vi "Initiate TS.vi"(8 "error in":errorcluster, 11 "HTS Test Stand in":refnum<class "HTS Test Stand.lvclass">) -> (0 "error out":errorcluster, 3 "HTS Test Stand out":refnum<class "HTS Test Stand.lvclass">)   [LabVIEW 2019, in "Test Stands.lvlib" / "HTS Test Stand.lvclass"]
uses:
  HTS Test Stand.lvclass
  DAC/HTS/Vacum Valve/DAC Vacum Valve.lvclass
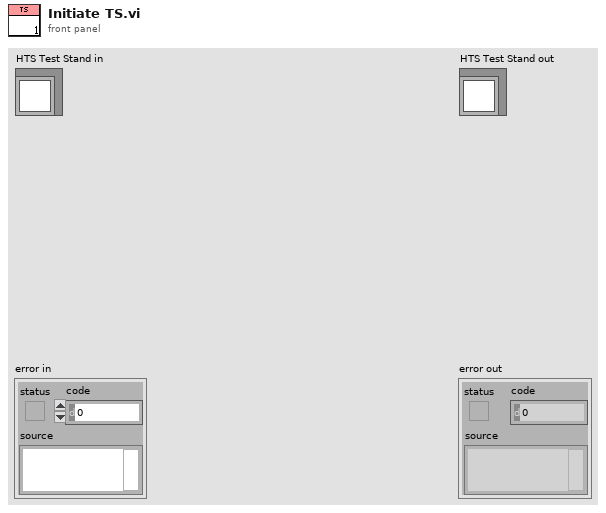
[diagram p1: front panel]
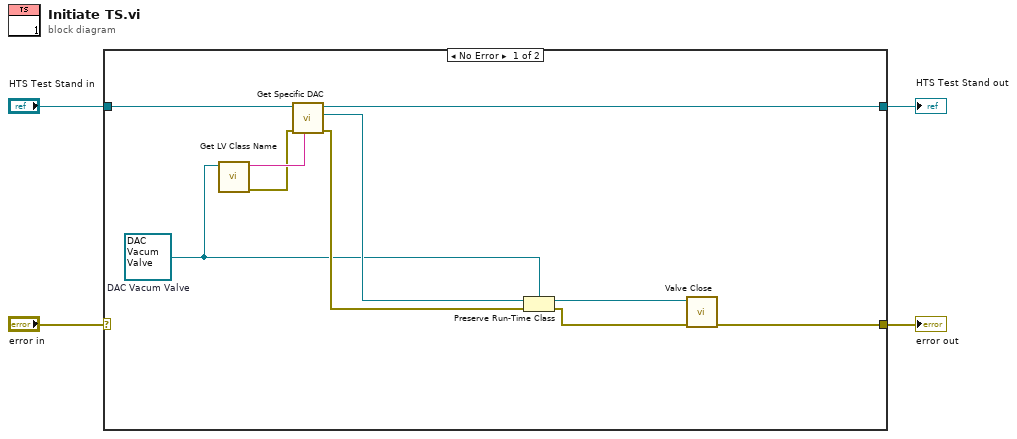
[diagram p0: block diagram]
diagram:
  n1 = case shown="No Error" "error in" {
    selector: "error in" -> [_ w16]
    tunnel: [w14 w16] -> w4
    tunnel: [w12 w15] -> w3
    tunnel: "HTS Test Stand in" -> [w13 w15]
    frame No Error {
      w7 = refnum<class "DAC Vacum Valve.lvclass"> refnum  # DAC Vacum Valve
      n2 = call <vilib>:"Get LV Class Name.vi"("object"=w7) -> ("error out"=w9:errorcluster, "class name"=w11:string)  [unwired: 9 in]
      n3 = call-dynamic "Get Specific DAC.vi"("DAC Class Name"=w11, "error in"=w9, "Generic Test Stand in"=w13) -> ("error out"=w8:errorcluster, "DAC"=w10:refnum<class "DAC.lvclass">, "Generic Test Stand out"=w12:refnum<class "HTS Test Stand.lvclass">)  [unwired: 6 in]
      n4 = Preserve Run-Time Class(object in=w10, error in=w8, 2:w7) -> (object out=w6:refnum<class "DAC Vacum Valve.lvclass">, error out=w5:errorcluster)
      n5 = call "Valve Close.vi"("error in (no error)"=w5, "DAC Vacum Valve in"=w6) -> ("error out"=w14:errorcluster)  [unwired: 8 in, 1 out]
    }
    frame Error {
    }
  }
  "error out" <- w4
  "HTS Test Stand out" <- w3
